vi "ConfigParams - Set - OperationalModes.vi"(7 "CellInhibitEnable":bool, 8 "error in (no error)":errorcluster, 11 "Ethernet in":refnum<class "ENET_BS1201.lvclass">) -> (0 "error out":errorcluster, 3 "Ethernet out":refnum<class "ENET_BS1201.lvclass">)   [LabVIEW 2021, in "BS120x Driver.lvlib" / "ENET_BS1201.lvclass"]
doc: "Configure the Cell Inhibit Enable function. Unit must be restarted to take effect."
uses:
  ENET_BS1201.lvclass
panel:
  # "[OperationalModes]\nCellInhibitEnable = False"
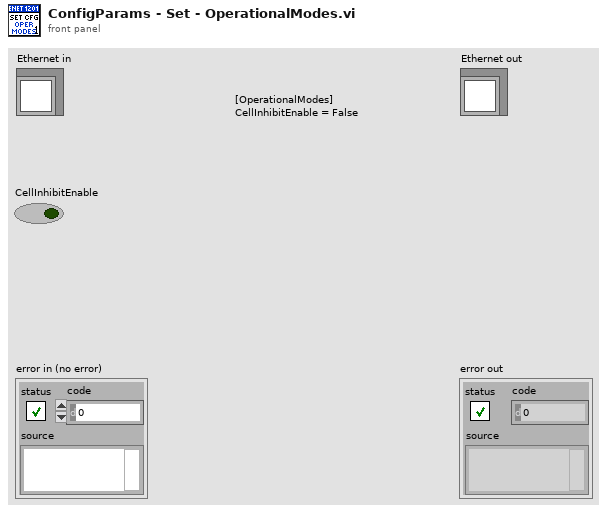
[diagram p1: front panel]
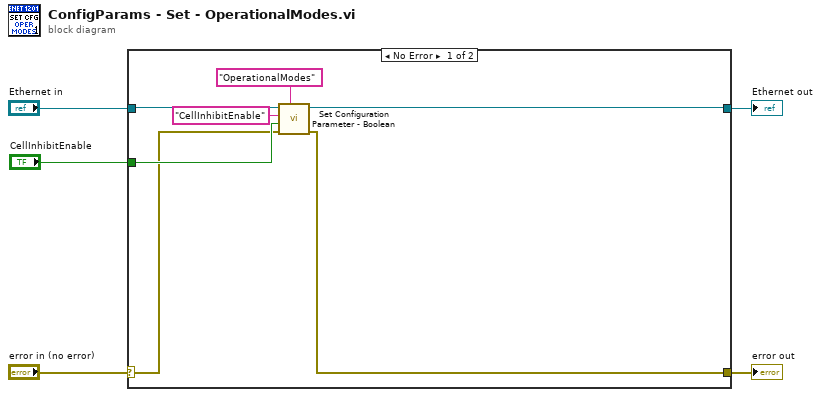
[diagram p0: block diagram]
diagram:
  n1 = case shown="No Error" "error in (no error)" {
    selector: "error in (no error)" -> [w8 w14]
    tunnel: [w6 w14] -> w4
    tunnel: [w7 w13] -> w2
    tunnel: "Ethernet in" -> [w12 w13]
    tunnel: "CellInhibitEnable" -> [w10 _]
    frame No Error {
      n2 = call-dynamic "Set Configuration Parameter - Boolean.vi"("Section"="OperationalModes", "error in (no error)"=w8, "Value"=w10, "Key"="CellInhibitEnable", "Ethernet in"=w12) -> ("error out"=w6:errorcluster, "Ethernet out"=w7:refnum<class "ENET_BS1201.lvclass">)  [unwired: 5 in]
    }
    frame Error {
    }
  }
  "error out" <- w4
  "Ethernet out" <- w2
